vi "Set properties.vi"(8 "error in (no error)":errorcluster, 11 "Two Lockins in":refnum<class "Two Lockins.lvclass">) -> (0 "error out":errorcluster, 3 "Two Lockins out":refnum<class "Two Lockins.lvclass">)   [LabVIEW 2017, in "Two Lockins.lvclass"]
uses:
  Two Lockins.lvclass
  Two Lockins.lvclass/Two Lockins.ctl
  Lockin/sr830/SR830.lvlib
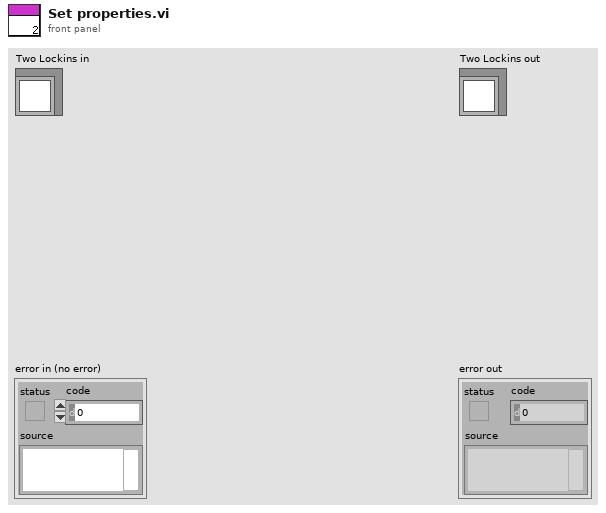
[diagram p1: front panel]
types:
  T1 = typedef "Lockin SR830.lvclass/Sensitivity.ctl" = u16
  T2 = typedef "SR830.lvlib/Tau.ctl" = u16
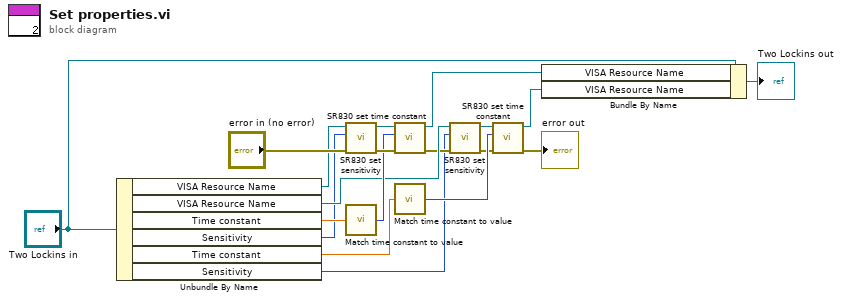
[diagram p0: block diagram]
diagram:
  n1 = Unbundle By Name("Two Lockins in") -> ("VISA Resource Name"=w10:refnum<visa-resource-name>, "VISA Resource Name"=w9:refnum<visa-resource-name>, "Time constant"=w12:dbl[unit], "Sensitivity"=w3:T1, "Time constant"=w5:dbl[unit], "Sensitivity"=w6:T1)
  n2 = call "SR830 set sensitivity.vi"("error in (no error)"="error in (no error)", "Sensitivity"=w3, "VISA resource name"=w10) -> ("error out"=w18:errorcluster, "VISA resource name out"=w19:refnum<visa-resource-name>)  [unwired: 7 in]
  n3 = call "Match time constant to value.vi"("Time constant"=w12) -> ("Tau"=w17:T2)
  n4 = call "SR830 set time constant.vi"("error in (no error)"=w18, "Tau"=w17, "VISA resource name"=w19) -> ("error out"=w8:errorcluster, "VISA resource name out"=w1:refnum<visa-resource-name>)  [unwired: 7 in]
  n5 = call "Match time constant to value.vi"("Time constant"=w5) -> ("Tau"=w15:T2)
  n6 = call "SR830 set sensitivity.vi"("error in (no error)"=w8, "Sensitivity"=w6, "VISA resource name"=w9) -> ("error out"=w14:errorcluster, "VISA resource name out"=w13:refnum<visa-resource-name>)  [unwired: 7 in]
  n7 = call "SR830 set time constant.vi"("error in (no error)"=w14, "Tau"=w15, "VISA resource name"=w13) -> ("error out"=→"error out":errorcluster, "VISA resource name out"=w2:refnum<visa-resource-name>)  [unwired: 7 in]
  n8 = Bundle By Name(cluster="Two Lockins in", "VISA Resource Name"=w1, "VISA Resource Name"=w2) -> (→"Two Lockins out":refnum<class "Two Lockins.lvclass">)
